vi "TransportTeardown.vi"(11 "EventRef":refnum<event-registration>) -> (1 "UnhandledMsgs":refnum<class "Msg.lvclass">[](array[class]), 2 "UnhandledMsgAttribs":T1[](array[typedef]) {"Listen Absolute Time" format="%<%x %.3X>T"; "Tell Absolute Time" format="%<%x %.3X>T"}, 3 "EventRef":refnum<event-registration>)   [LabVIEW 2020, in "jettl.lvlib"]
uses:
  jettl.lvlib
  Msg/Msg.lvclass
  Origin.ctl
  Lifecycle.ctl
  Msg Attribs.ctl
  Msg.ctl
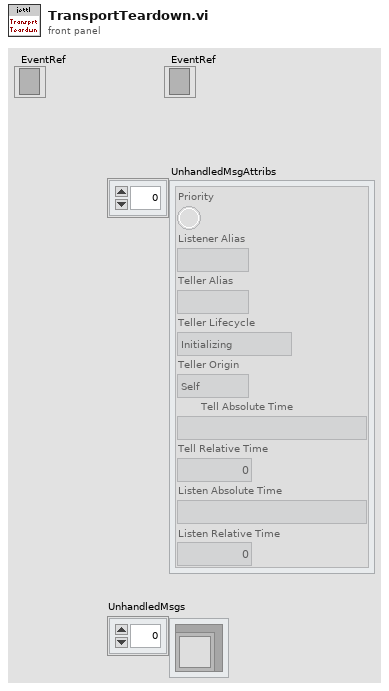
[diagram p1: front panel]
types:
  T1 = typedef "jettl.lvlib/Msg Attribs.ctl" = cluster{"Priority":bool, "Listener Alias":string, "Teller Alias":string, "Teller Lifecycle":T2, "Teller Origin":T3, "Tell Absolute Time":timestamp, "Tell Relative Time":dbl, "Listen Absolute Time":timestamp, "Listen Relative Time":dbl}
  T2 = typedef "jettl.lvlib/Lifecycle.ctl" = enum16{"Initializing", "Setting Up", "Starting", "Running", "Stopping", "Tearing Down", "Terminated"}
  T3 = typedef "jettl.lvlib/Origin.ctl" = enum16{"Self", "Parent", "Child"}
  T4 = typedef "jettl.lvlib/MsgAttribs.ctl" = cluster{"Priority":bool, "MsgExecuteType":T5, "ListenerAlias":string, "TellerAlias":string, "Origin":T3, "Lifecycle":T6, "AbsoluteTime":timestamp, "RelativeTime":dbl, "Metadata":refnum<class "Metadata.lvclass">}
  T5 = typedef "jettl.lvlib/MsgExecuteType.ctl" = enum16{"Tell", "Call"}
  T6 = typedef "jettl.lvlib/Lifecycle.ctl" = enum16{"Initializing", "SettingUp", "Starting", "Running", "Stopping", "TearingDown", "Terminated"}
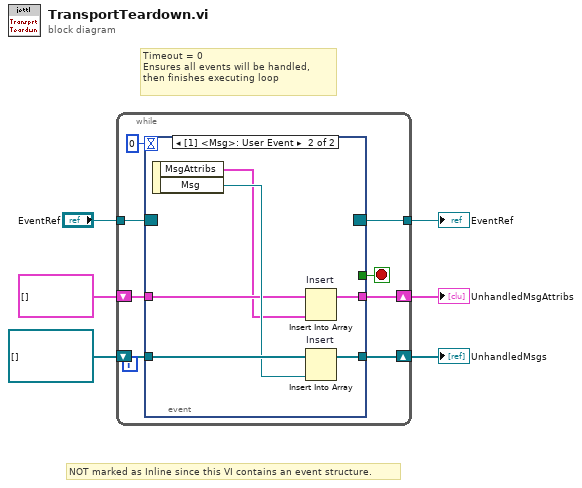
[diagram p0: block diagram]
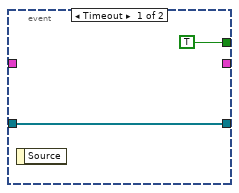
[diagram p2: hidden frame]
diagram:
  # "NOT marked as Inline since this VI contains an event structure."
  # "Timeout = 0\nEnsures all events will be handled, then finishes executing loop"
  n1 = while {
    shift-right: [w13] -> w4
    shift-left: refnum<class "Msg.lvclass">[] [] -> [w14]
    tunnel: "EventRef" -> [w12]
    tunnel: [w9] -> w3
    shift-right: [w8] -> w1
    shift-left: T1[] [] -> [w7]
    stop <- w11 stop-if-true
    n2 = event shown="[1] <Msg>: User Event" {
      selector: w12 -> [_ _]
      dyn-events: [_ _] -> w9
      timeout: 0 -> [_ _]
      tunnel: w14 -> [w16 w22]
      tunnel: [w16 w21] -> w13
      tunnel: [TRUE _] -> w11
      tunnel: [_ w18] -> w8
      tunnel: w7 -> [_ w19]
      event Timeout {
        n3 = event-data() -> ()  [unwired: 1 in, 1 out]
      }
      event User Event {
        n4 = event-data() -> ("MsgAttribs"=w17:T4, "Msg"=w20:refnum<class "Msg.lvclass">)  [unwired: 1 in]
        n5 = Insert Into Array "Insert"(array=w19, new element=w17) -> (w18:T1[])  [unwired: 1 in]
        n6 = Insert Into Array "Insert"(array=w22, new element=w20) -> (w21:refnum<class "Msg.lvclass">[])  [unwired: 1 in]
      }
    }
  }
  "UnhandledMsgs" <- w4
  "EventRef" <- w3
  "UnhandledMsgAttribs" <- w1
